vi "Test Pump Connection.vi"() -> ()   [LabVIEW 2018, in "VICI M6 M50 Party Mode.lvlib"]
uses:
  VICI M6 M50 Party Mode.lvlib
  <vilib>/Instr/_visa.llb/VISA Configure Serial Port (Instr).vi
panel:
  in  "stop":bool
  in  "Enum":T1(ring)=enum."Save"
  out "read buffer 4":string
  out "Bytes at Port 5":u32
  out "String 2":string
  out "Bytes at Port 4":u32
  out "read buffer 3":string
  in  "Pump Letter":string
  out "error out":errorcluster
  out "VISA resource name out":refnum<visa-resource-name>
  in  "VISA resource name":refnum<visa-resource-name>
  in  "error in (no error)":errorcluster
  # "Copyright\\A9\\s2010\\sSchneider\\sElectric\\sMotion\\sUSA\\r\\n"
  # "Copyright© 2010 Schneider Electric Motion USA"
  # "A\\s=\\s1000000\\r\\n"
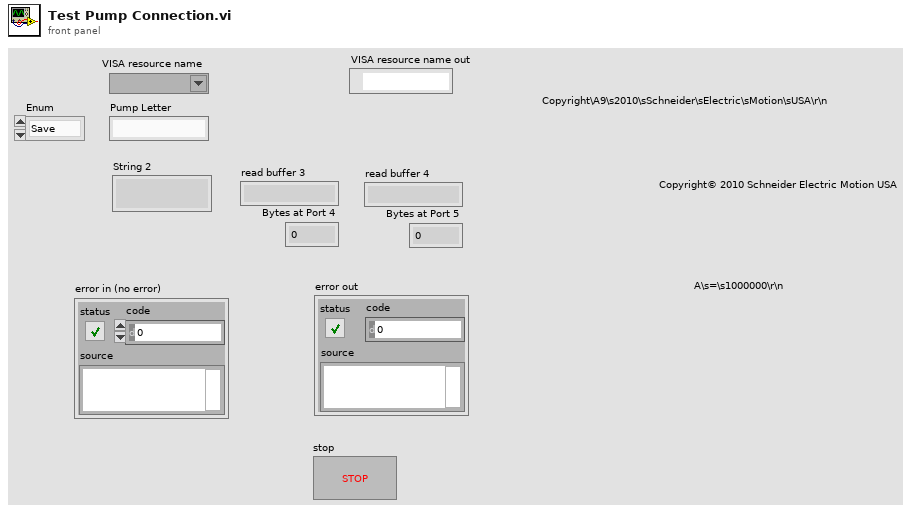
[diagram p1: front panel]
types:
  T1 = enum16{"Default", "Letter", "Save", "Party", "Test", "Error Check", "Error Print"}
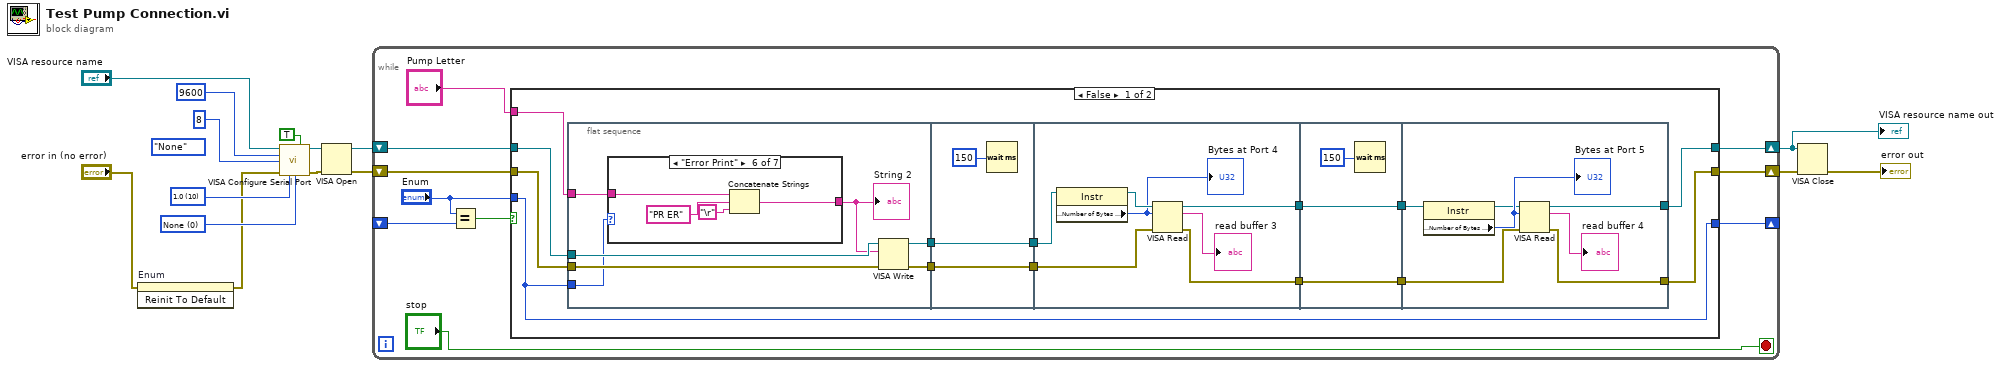
[diagram p0: block diagram]
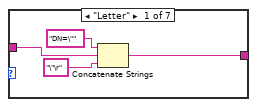
[diagram p2: hidden frame]
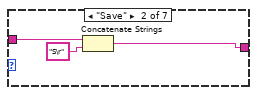
[diagram p3: hidden frame]
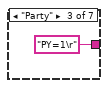
[diagram p4: hidden frame]
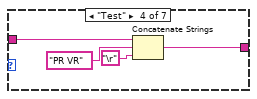
[diagram p5: hidden frame]
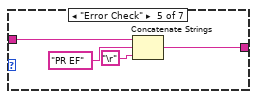
[diagram p6: hidden frame]
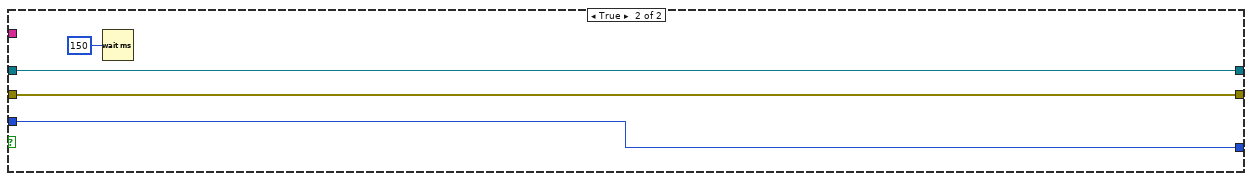
[diagram p8: hidden frame]
diagram:
  w8 = u16 0 items=["None", "XON/XOFF", "RTS/CTS", "XON/XOFF & RTS/CTS", "DTR/DSR", "XON/XOFF & DTR/DSR"] ("flow control (0:none)")
  w9 = u16 10 items=["1.0"=10, "1.5"=15, "2.0"=20] ("stop bits (10: 1 bit)")
  (unwired) enum16{"None", "Odd", "Even", "Mark", "Space"}."None" ("parity (0:none)")
  n1 = invoke on="Enum" class="Enum (strict)" method="Reinit To Default"(error in="error in (no error)") -> (error out=w1:errorcluster)  [unwired: 2 in, 2 out]
  n2 = call-poly "VISA Configure Serial Port"("VISA resource name"="VISA resource name", "Enable Termination\nChar (T)"=TRUE ("Enable Termination\nChar (T)"), "baud rate (9600)"=u32 9600, "data bits (8)"=u16 8, "error in (no error)"=w1, "stop bits (10: 1 bit)"=w9, "flow control (0:none)"=w8) -> ("VISA resource name out"=w14:refnum<visa-resource-name>, "error out"=w13:errorcluster)  [unwired: 7 in]
  n3 = VISA Open(error in (no error)=w13, VISA resource name=w14) -> (VISA resource name=w6:refnum<visa-resource-name>, error out=w7:errorcluster)  [unwired: 3 in]
  n4 = while {
    shift-right: [w23] -> w4
    shift-left: w7 -> [w25]
    shift-right: [w22] -> w3
    shift-left: w6 -> [w24]
    shift-right: [w20] -> _
    shift-left: _ -> [w16]
    stop <- "stop" stop-if-true
    n5 = Equal?(x="Enum", y=w16) -> (x = y?=w19:bool)
    n6 = case shown="False" w19 {
      tunnel: w25 -> [w31 w88]
      tunnel: w24 -> [w30 w89]
      tunnel: "Pump Letter" -> [w29 _]
      tunnel: [w28 w88] -> w23
      tunnel: [w27 w89] -> w22
      tunnel: "Enum" -> [w26 w90]
      tunnel: [w26 w90] -> w20
      frame False {
        n7 = flat-sequence {
          tunnel: w30 -> [w46]
          tunnel: w29 -> [w45]
          tunnel: w31 -> [w44]
          tunnel: [w43] -> w39
          tunnel: [w42] -> w38
          tunnel: w26 -> [w40]
          tunnel: [w70] -> w37
          tunnel: w39 -> [w70]
          tunnel: [w69] -> w36
          tunnel: w38 -> [w69]
          tunnel: w37 -> [w74]
          tunnel: w36 -> [w73]
          tunnel: [w72] -> w35
          tunnel: [w71] -> w34
          tunnel: w35 -> [w80]
          tunnel: [w80] -> w33
          tunnel: w34 -> [w79]
          tunnel: [w79] -> w32
          tunnel: w33 -> [w84]
          tunnel: w32 -> [w83]
          tunnel: [w82] -> w27
          tunnel: [w81] -> w28
          frame #0 {
            n8 = case shown="\"Error Print\"" w40 {
              tunnel: w45 -> [w48 w53 _ w55 w59 w63 w67]
              tunnel: [w47 w51 "PY=1\r" ("string") w56 w60 w64 w67] -> w41
              frame "Letter" {
                n9 = Concatenate Strings("DN=\"" ("string"), w48, "\"\r" ("string")) -> (w47:string)
              }
              frame "Save" {
                n10 = Concatenate Strings(w53, "S\r" ("string")) -> (w51:string)
              }
              frame "Party" {
              }
              frame "Test" {
                n11 = Concatenate Strings(w55, "PR VR" ("string"), "\r") -> (w56:string)
              }
              frame "Error Check" {
                n12 = Concatenate Strings(w59, "PR EF" ("string"), "\r") -> (w60:string)
              }
              frame "Error Print" {
                n13 = Concatenate Strings(w63, "PR ER" ("string"), "\r") -> (w64:string)
              }
              frame "Default", Default {
              }
            }
            "String 2" <- w41
            n14 = VISA Write(VISA resource name=w46, write buffer=w41, error in (no error)=w44) -> (VISA resource name out=w43:refnum<visa-resource-name>, error out=w42:errorcluster)  [unwired: 1 out]
          }
          frame #1 {
            n15 = Wait (ms)(milliseconds to wait=u32 150) -> ()  [unwired: 1 out]
          }
          frame #2 {
            n16 = property class="Instr"(reference=w74) -> (reference out=w77:refnum<visa-resource-name>, "Serial Settings:Number of Bytes at Serial Port"=w76:u32)  [unwired: 1 in, 1 out]
            "Bytes at Port 4" <- w76
            n17 = VISA Read(VISA resource name=w77, byte count=w76, error in (no error)=w73) -> (VISA resource name out=w72:refnum<visa-resource-name>, read buffer=→"read buffer 3":string, error out=w71:errorcluster)  [unwired: 1 out]
          }
          frame #3 {
            n18 = Wait (ms)(milliseconds to wait=u32 150) -> ()  [unwired: 1 out]
          }
          frame #4 {
            n19 = property class="Instr"(reference=w84) -> (reference out=w85:refnum<visa-resource-name>, "Serial Settings:Number of Bytes at Serial Port"=w86:u32)  [unwired: 1 in, 1 out]
            "Bytes at Port 5" <- w86
            n20 = VISA Read(VISA resource name=w85, byte count=w86, error in (no error)=w83) -> (VISA resource name out=w82:refnum<visa-resource-name>, read buffer=→"read buffer 4":string, error out=w81:errorcluster)  [unwired: 1 out]
          }
        }
      }
      frame True {
        n21 = Wait (ms)(milliseconds to wait=u32 150) -> ()  [unwired: 1 out]
      }
    }
  }
  "VISA resource name out" <- w3
  n22 = VISA Close(VISA resource name=w3, error in (no error)=w4) -> (error out=→"error out":errorcluster)
